vi "PNAinit.vi"(2 "Error In (no error)":errorcluster, 3 "Meas":T2, 4 "PNA Config":T1={"Sweep Type"=0, "Sweep Gen Type"=0, "Sweep Points"=1001, "Bandwidth (Hz)"=1000.0, "Center Freq (Hz)"=6000000000.0, "Span Freq (Hz)"=4000000000.0, "Power Level (dBm)"=-70.0, "Average Count"=1, "Electrical Delay (s)"=0.0} {"Electrical Delay (s)" format="%.6p"; "Power Level (dBm)" format="%.2p"; "Span Freq (Hz)" format="%.6p"; "Center Freq (Hz)" format="%.6p"; "Bandwidth (Hz)" format="%.2p"; "Sweep Gen Type" items=["Analog", "Stepped"]; "Sweep Type" items=["Linear Frequency", "Log Frequency", "Power Sweep", "CW Time"]}, 5 "VISA session":refnum<visa-resource-name>) -> (0 "Error Out":errorcluster, 1 "dup VISA session":refnum<visa-resource-name>)   [LabVIEW 2017]
uses:
  <instrlib>/Agilent PNA Series/Agilent PNA Series.lvlib
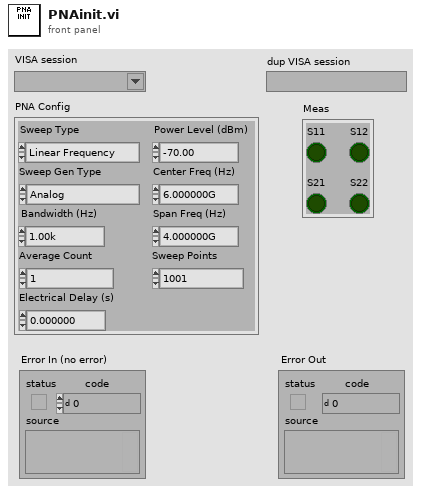
[diagram p1: front panel]
types:
  T1 = cluster{"Sweep Type":i32, "Sweep Gen Type":i32, "Sweep Points":i32, "Bandwidth (Hz)":dbl, "Center Freq (Hz)":dbl, "Span Freq (Hz)":dbl, "Power Level (dBm)":dbl, "Average Count":i32, "Electrical Delay (s)":dbl}
  T2 = cluster{"S11":bool, "S12":bool, "S21":bool, "S22":bool}
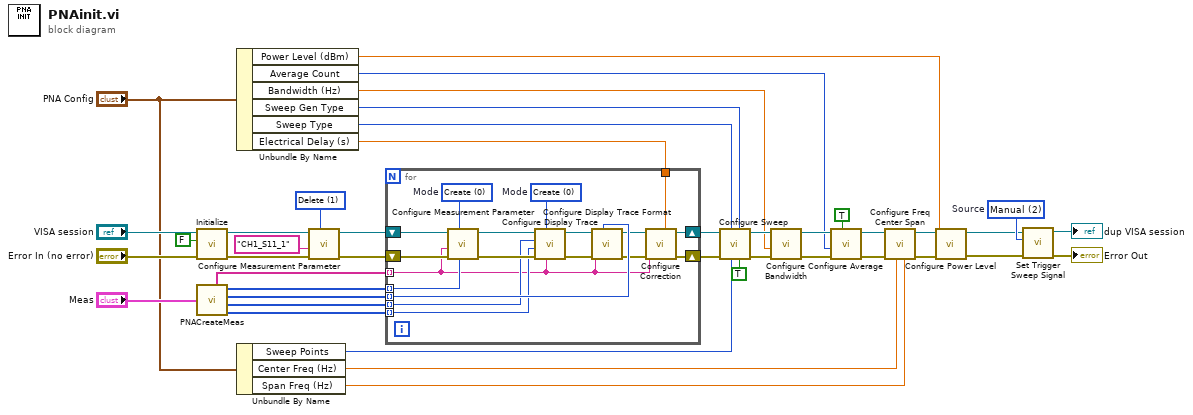
[diagram p0: block diagram]
diagram:
  w31 = u16 1 items=["Create", "Delete", "Select"] ("Mode (0: Create)")
  w39 = u16 2 items=["Immediate", "External", "Manual"]  # Source
  n1 = call <instrlib>:"Initialize.vi"("error in (no error)"="Error In (no error)", "ID Query (T: Check)"=FALSE, "Instrument Resource Name"="VISA session") -> ("error out"=w34:errorcluster, "dup VISA session"=w35:refnum<visa-resource-name>)  [unwired: 7 in]
  n2 = call "PNACreateMeas.vi"("Meas in"="Meas") -> ("Disp traces"=w14:i32[], "Disp windows"=w15:i32[], "Disp format"=w16:i32[], "Meas types"=w18:i32[], "Meas names"=w17:string[])
  n3 = Unbundle By Name("PNA Config") -> ("Power Level (dBm)"=w19:dbl, "Average Count"=w9:i32, "Bandwidth (Hz)"=w29:dbl, "Sweep Gen Type"=w28:i32, "Sweep Type"=w27:i32, "Electrical Delay (s)"=w7:dbl)
  n4 = Unbundle By Name("PNA Config") -> ("Sweep Points"=w26:i32, "Center Freq (Hz)"=w25:dbl, "Span Freq (Hz)"=w24:dbl)
  n5 = call <instrlib>:"Configure Measurement Parameter.vi"("Mode (0: Create)"=w31, "Error In (no error)"=w34, "Measurement Name (MY_MEAS)"="CH1_S11_1", "VISA Resource Name"=w35) -> ("Error Out"=w32:errorcluster, "VISA Resource Name Out"=w33:refnum<visa-resource-name>)  [unwired: 6 in]
  n6 = for {
    shift-right: [w47] -> w36
    shift-left: w32 -> [w59]
    shift-right: [w48] -> w37
    shift-left: w33 -> [w58]
    tunnel: w17 -> [w43] mode=indexing
    tunnel: w18 -> [w54] mode=indexing
    tunnel: w16 -> [w51] mode=indexing
    tunnel: w15 -> [w50] mode=indexing
    tunnel: w14 -> [w49] mode=indexing
    tunnel: w7 -> [w44]
    w57 = u16 0 items=["Create", "Delete"]  # Mode
    w60 = u16 0 items=["Create", "Delete", "Select"]  # Mode
    n7 = call <instrlib>:"Configure Measurement Parameter.vi"("Measurement Type (0: S11)"=w54, "Mode (0: Create)"=w60, "Error In (no error)"=w59, "Measurement Name (MY_MEAS)"=w43, "VISA Resource Name"=w58) -> ("Error Out"=w55:errorcluster, "VISA Resource Name Out"=w56:refnum<visa-resource-name>)  [unwired: 5 in]
    n8 = call <instrlib>:"Configure Display Trace.vi"("Measurement Name (MY_MEAS)"=w43, "Mode (0: Create)"=w57, "Error In (no error)"=w55, "Display Trace (1)"=w49, "Display Window (1)"=w50, "VISA Resource Name"=w56) -> ("Error Out"=w52:errorcluster, "VISA Resource Name Out"=w53:refnum<visa-resource-name>)  [unwired: 4 in]
    n9 = call <instrlib>:"Configure Display Trace Format.vi"("Display Trace Format (0: Magnitude Logarithmic)"=w51, "Error In (no error)"=w52, "Measurement Name (MY_MEAS)"=w43, "VISA session"=w53) -> ("Error Out"=w45:errorcluster, "dup VISA session"=w46:refnum<visa-resource-name>)  [unwired: 6 in]
    n10 = call <instrlib>:"Configure Correction.vi"("Correction Electrical Delay (0.0)"=w44, "Error In (no error)"=w45, "Measurement Name (MY_MEAS)"=w43, "VISA session"=w46) -> ("Error Out"=w47:errorcluster, "dup VISA session"=w48:refnum<visa-resource-name>)  [unwired: 6 in]
  }
  n11 = call <instrlib>:"Configure Sweep.vi"("Sweep Time Auto (T: On)"=TRUE ("Sweep Time Auto"), "Sweep Gen Type (0: Analog)"=w28, "Sweep Points (201)"=w26, "Sweep Type (0: Linear Frequency)"=w27, "Error In (no error)"=w36, "VISA session"=w37) -> ("Error Out"=w41:errorcluster, "dup VISA session"=w42:refnum<visa-resource-name>)  [unwired: 4 in]
  n12 = call <instrlib>:"Configure Bandwidth.vi"("Error In (no error)"=w41, "Bandwidth (20.0E+3)"=w29, "VISA session"=w42) -> ("Error Out"=w13:errorcluster, "dup VISA session"=w11:refnum<visa-resource-name>)  [unwired: 7 in]
  n13 = call <instrlib>:"Configure Average.vi"("Average State (F: Off)"=TRUE, "Error In (no error)"=w13, "Average Count (1)"=w9, "VISA Resource Name"=w11) -> ("Error Out"=w12:errorcluster, "VISA Resource Name Out"=w10:refnum<visa-resource-name>)  [unwired: 6 in]
  n14 = call <instrlib>:"Configure Freq Center Span.vi"("Span Freq (2.9997 E+9)"=w24, "Center Freq (1.50015 E+9)"=w25, "Error In (no error)"=w12, "VISA session"=w10) -> ("Error Out"=w20:errorcluster, "dup VISA session"=w23:refnum<visa-resource-name>)  [unwired: 6 in]
  n15 = call <instrlib>:"Configure Power Level.vi"("Error In (no error)"=w20, "Power Level (0.0)"=w19, "VISA Resource Name"=w23) -> ("Error Out"=w21:errorcluster, "VISA Resource Name Out"=w22:refnum<visa-resource-name>)  [unwired: 7 in]
  n16 = call <instrlib>:"Set Trigger Sweep Signal.vi"("Error In (no error)"=w21, "Source (0: Immediate)"=w39, "VISA session"=w22) -> ("Error Out"=→"Error Out":errorcluster, "dup VISA session"=→"dup VISA session":refnum<visa-resource-name>)  [unwired: 7 in]
